vi "Memory.Pointer.U64.New.vi"(8 "error in (no error)":errorcluster) -> (0 "error out":errorcluster, 3 "U64 Pointer":refnum<class "Memory.Pointer.U64.lvclass">)   [LabVIEW 2016, in "LabVIEW Memory Manager.lvlib" / "Memory.Pointer.U64.lvclass"]
uses:
  Memory.Pointer.U64.lvclass
  C:/Users/Ryan/Documents/Git/Sourcetree/LabVIEW-Memory-Manager/Source/Library/Classes/Pointer/Memory.Pointer.Void.lvclass
  Pointer/Memory.Pointer.Void.lvclass/Memory.Pointer.Void.ctl
  Pointer/Methods/Memory.Pointer.Set Address.vi
  Pointer/Methods/Memory.Pointer.Set Size.vi
  Pointer/Memory.Pointer.Void.lvclass
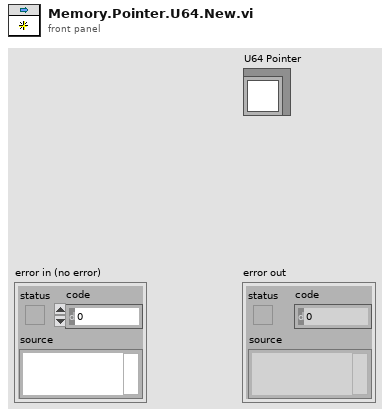
[diagram p1: front panel]
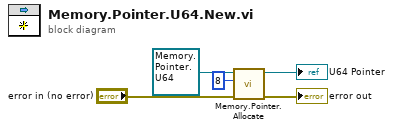
[diagram p0: block diagram]
diagram:
  n1 = call "Memory.Pointer.Allocate.vi"("error in (no error)"="error in (no error)", "size"=u64 8, "Pointer in"=refnum<class "Memory.Pointer.U64.lvclass"> refnum ("LabVIEW Memory Manager.lvlib:DBL Pointer")) -> ("error out"=→"error out":errorcluster, "Pointer out"=→"U64 Pointer":refnum<class "Memory.Pointer.U64.lvclass">)  [unwired: 6 in, 1 out]
